vi "Proceed.vi"(7 "component is ready (Y)":bool=TRUE, 8 "error in (no error)":errorcluster, 10 "ProceedMessage":refnum<class "ProceedMessage.lvclass">, 11 "Thorcam in":refnum<class "Thorcam.lvclass">) -> (0 "error out":errorcluster, 2 "all observers are ready?":bool, 3 "Thorcam out":refnum<class "Thorcam.lvclass">)   [LabVIEW 2012, in "Thorcam.lvclass"]
doc: "The Proceed method is used to check if your component is ready. Also it checks if the observers are ready. When the observers and the component are ready, it sends the proceed to its observee. If it's the highest observee, it distributes a stop command."
uses:
  Thorcam.lvclass
  <vilib>/Distrio/Murmex/ProceedMessage/ProceedMessage.lvclass
  Thorcam.lvclass/Thorcam.ctl
  <vilib>/Distrio/Murmex/Murmex/Murmex.lvclass
panel:
  # "This method is called when the PROCEED\ntrigger is sent. \n\nOverride this method when your component needs to\nrespond to this trigger. \n\nCall parent for proper implementation"
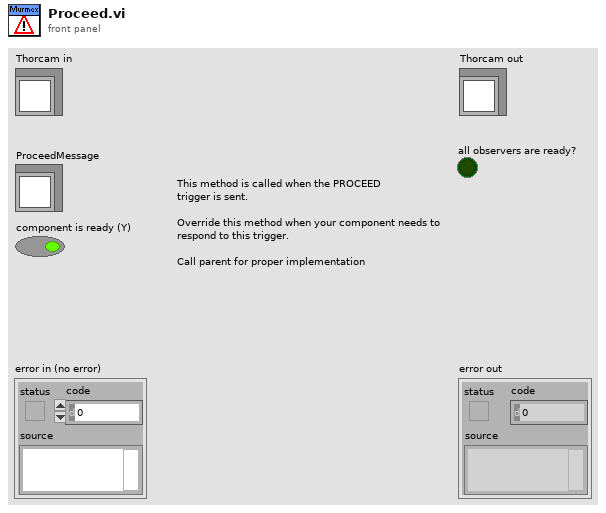
[diagram p1: front panel]
types:
  T1 = typedef "Thorcam.lvclass/current task.ctl" = enum16{"Camera", "Phase Comparison", "Pre-Tomo"}
  T2 = typedef "Thorcam.lvclass/imaging mode.ctl" = enum16{"free run mode", "single frame"}
  T3 = typedef "IMAQ Image.ctl" = refnum<image>
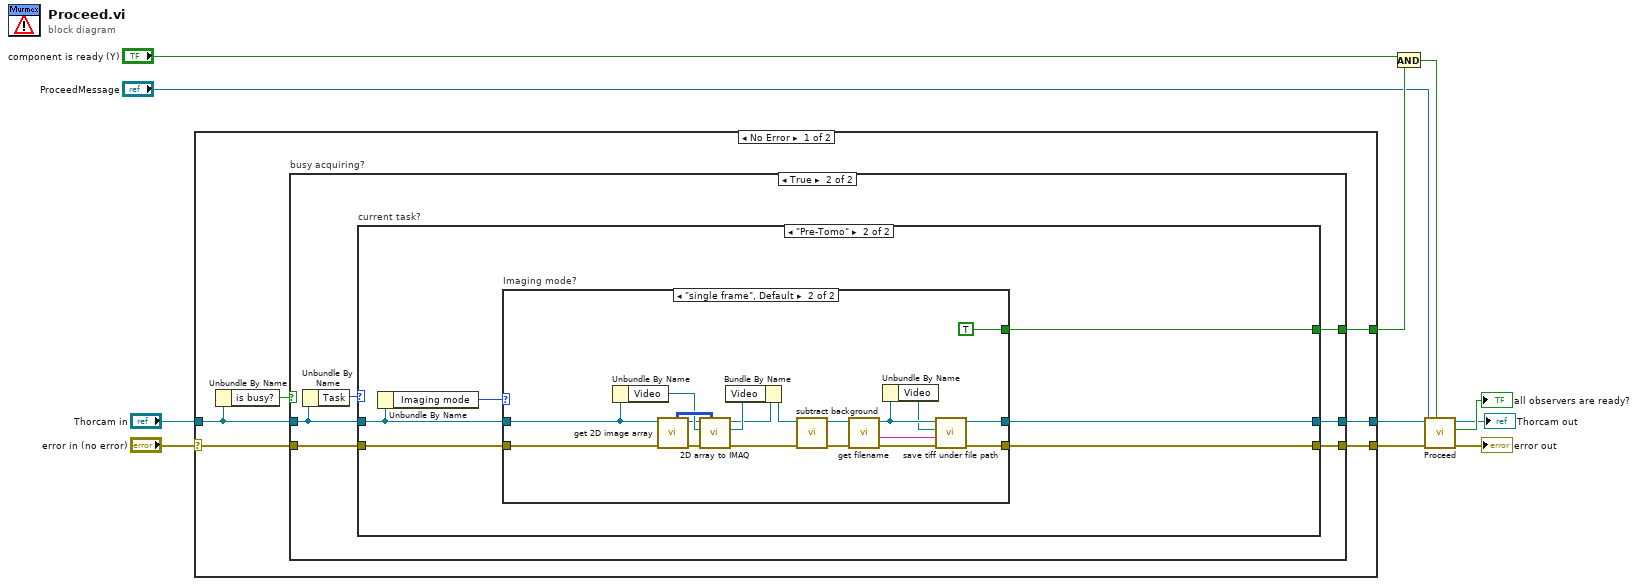
[diagram p0: block diagram]
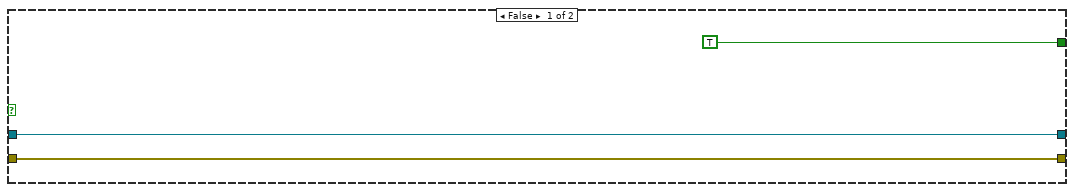
[diagram p2: hidden frame]
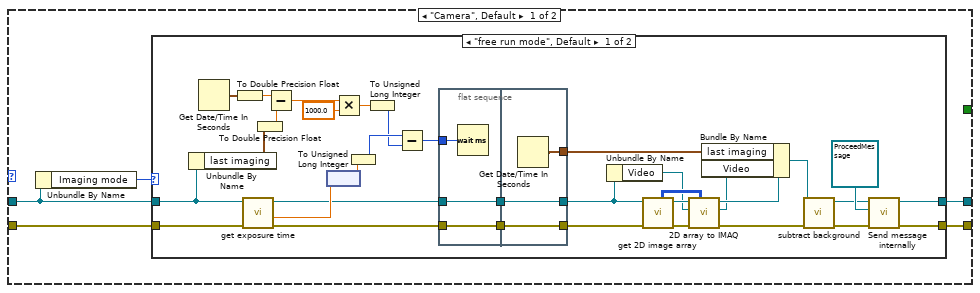
[diagram p3: hidden frame]
diagram:
  n1 = case shown="No Error" "error in (no error)" {
    selector: "error in (no error)" -> [w17 w102]
    tunnel: [w16 w102] -> w8
    tunnel: "Thorcam in" -> [w14 w101]
    tunnel: [w15 w101] -> w6
    tunnel: [w12 _] -> w3
    frame No Error {
      n2 = Unbundle By Name(w14) -> ("is busy?"=w13:bool)
      n3 = case "busy acquiring?" shown="True" w13 {
        tunnel: w17 -> [w20 w26]
        tunnel: [w20 w25] -> w16
        tunnel: [w19 w24] -> w15
        tunnel: w14 -> [w19 w23]
        tunnel: [TRUE w21] -> w12
        frame False {
        }
        frame True {
          n4 = Unbundle By Name(w23) -> ("Task"=w22:T1)
          n5 = case "current task?" shown="\"Pre-Tomo\"" w22 {
            tunnel: w26 -> [w31 w79]
            tunnel: [w30 w76] -> w25
            tunnel: [w27 w75] -> w24
            tunnel: w23 -> [w29 w78]
            tunnel: [_ w74] -> w21
            frame "Camera", Default {
              n6 = Unbundle By Name(w29) -> ("Imaging mode"=w28:T2)
              n7 = case shown="\"free run mode\", Default" w28 {
                tunnel: w31 -> [w42 w73]
                tunnel: [w45 w73] -> w30
                tunnel: w29 -> [w43 w72]
                tunnel: [w46 w72] -> w27
                frame "free run mode", Default {
                  n8 = Unbundle By Name(w43) -> ("last imaging"=w51:timestamp)
                  n9 = Get Date/Time In Seconds() -> (seconds since 1Jan1904=w52:timestamp)
                  n10 = To Double Precision Float(number=w52) -> (double precision float=w50:dbl)
                  n11 = call-dynamic "get exposure time.vi"("error in (no error)"=w42, "Thorcam in"=w43) -> ("error out"=w38:errorcluster, "exposure time"=w62:dbl[unit], "Thorcam out"=w36:refnum<class "Thorcam.lvclass">)  [unwired: 7 in]
                  n12 = To Double Precision Float(number=w51) -> (double precision float=w49:dbl)
                  n13 = Subtract(x=w50, y=w49) -> (x-y=w48:dbl)
                  n14 = node(w62) -> (w61:dbl)
                  n15 = Multiply(x=w48, y=1000.0) -> (x*y=w41:dbl)
                  n16 = To Unsigned Long Integer(number=w61) -> (unsigned 32bit integer=w60:u32)
                  n17 = To Unsigned Long Integer(number=w41) -> (unsigned 32bit integer=w40:u32)
                  n18 = Subtract(x=w60, y=w40) -> (x-y=w35:u32)
                  n19 = flat-sequence {
                    tunnel: w38 -> [w68]
                    tunnel: w36 -> [w67]
                    tunnel: w35 -> [w66]
                    tunnel: [w68] -> w34
                    tunnel: [w67] -> w33
                    tunnel: [w70] -> w37
                    tunnel: [w71] -> w39
                    tunnel: w34 -> [w71]
                    tunnel: w33 -> [w70]
                    tunnel: [w69] -> w32
                    frame #0 {
                      n20 = Wait (ms)(milliseconds to wait=w66) -> ()  [unwired: 1 out]
                    }
                    frame #1 {
                      n21 = Get Date/Time In Seconds() -> (seconds since 1Jan1904=w69:timestamp)
                    }
                  }
                  n22 = Unbundle By Name(w37) -> ("Video"=w44:T3)
                  n23 = call-dynamic "get 2D image array.vi"("error in (no error)"=w39, "Thorcam in"=w37) -> ("error out"=w58:errorcluster, "Thorcam out"=w59:refnum<class "Thorcam.lvclass">, "image array out"=w57:u8[][])  [unwired: 7 in]
                  n24 = call-dynamic "2D array to IMAQ.vi"("Image Pixels (U8)"=w57, "error in (no error)"=w58, "Image"=w44, "Thorcam in"=w59) -> ("error out"=w54:errorcluster, "Image Out"=w55:T3, "Thorcam out"=w56:refnum<class "Thorcam.lvclass">)  [unwired: 5 in]
                  n25 = Bundle By Name(cluster=w56, "last imaging"=w32, "Video"=w55) -> (w53:refnum<class "Thorcam.lvclass">)
                  n26 = call-dynamic "subtract background.vi"("error in (no error)"=w54, "Thorcam in"=w53) -> ("error out"=w64:errorcluster, "Thorcam out"=w63:refnum<class "Thorcam.lvclass">)  [unwired: 8 in]
                  n27 = call <vilib>:"Send message internally.vi"("error in (no error)"=w64, "Message"=refnum<class "ProceedMessage.lvclass"> refnum ("Distrio Murmex 1.5:ProceedMessage"), "Murmex in"=w63) -> ("error out"=w45:errorcluster, "Murmex out"=w46:refnum<class "Thorcam.lvclass">)  [unwired: 7 in]
                }
                frame "single frame" {
                }
              }
            }
            frame "Pre-Tomo" {
              n28 = Unbundle By Name(w78) -> ("Imaging mode"=w77:T2)
              n29 = case "Imaging mode?" shown="\"single frame\", Default" w77 {
                tunnel: w79 -> [w81 w100]
                tunnel: w78 -> [w80 w99]
                tunnel: [w81 w92] -> w76
                tunnel: [w80 w86] -> w75
                tunnel: [_ TRUE] -> w74
                frame "free run mode" {
                }
                frame "single frame", Default {
                  n30 = Unbundle By Name(w99) -> ("Video"=w97:T3)
                  n31 = call-dynamic "get 2D image array.vi"("error in (no error)"=w100, "Thorcam in"=w99) -> ("error out"=w95:errorcluster, "Thorcam out"=w96:refnum<class "Thorcam.lvclass">, "image array out"=w98:u8[][])  [unwired: 7 in]
                  n32 = call-dynamic "2D array to IMAQ.vi"("Image Pixels (U8)"=w98, "error in (no error)"=w95, "Image"=w97, "Thorcam in"=w96) -> ("error out"=w93:errorcluster, "Image Out"=w94:T3, "Thorcam out"=w85:refnum<class "Thorcam.lvclass">)  [unwired: 5 in]
                  n33 = Bundle By Name(cluster=w85, "Video"=w94) -> (w84:refnum<class "Thorcam.lvclass">)
                  n34 = call-dynamic "subtract background.vi"("error in (no error)"=w93, "Thorcam in"=w84) -> ("error out"=w90:errorcluster, "Thorcam out"=w89:refnum<class "Thorcam.lvclass">)  [unwired: 8 in]
                  n35 = call-dynamic "get filename.vi"("error in (no error)"=w90, "Thorcam in"=w89) -> ("error out"=w88:errorcluster, "Filename"=w87:string, "Thorcam out"=w83:refnum<class "Thorcam.lvclass">)  [unwired: 7 in]
                  n36 = Unbundle By Name(w83) -> ("Video"=w82:T3)
                  n37 = call-dynamic "save tiff under file path.vi"("error in (no error)"=w88, "tiff name"=w87, "Image"=w82, "Thorcam in"=w83) -> ("error out"=w92:errorcluster, "Thorcam out"=w86:refnum<class "Thorcam.lvclass">)  [unwired: 6 in]
                }
              }
            }
          }
        }
      }
    }
    frame Error {
    }
  }
  n38 = And(x="component is ready (Y)", y=w3) -> (x .and. y?=w4:bool)
  n39 = call-parent "Proceed.vi"("component is ready (Y)"=w4, "error in (no error)"=w8, "ProceedMessage"="ProceedMessage", "Murmex in"=w6) -> ("error out"=→"error out":errorcluster, "all observers are ready?"=→"all observers are ready?":bool, "Murmex out"=→"Thorcam out":refnum<class "Thorcam.lvclass">)  [unwired: 5 in]
